vi "Remove Custom Device.vi"(8 "error in":errorcluster, 11 "Ballard ARINC 429 custom device":u64 format="%.0x") -> (0 "error out":errorcluster)   [LabVIEW 2020, in "Ballard ARINC 429 Scripting.lvlib"]
doc: "Removes the specified custom device from the system definition. Once the reference has been removed, it is no longer valid. This VI will return an error if called to remove an invalid reference."
uses:
  Ballard ARINC 429 Scripting.lvlib
  NationalInstruments.VeriStand.SystemDefinitionAPI
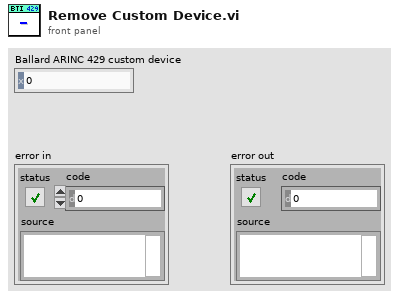
[diagram p1: front panel]
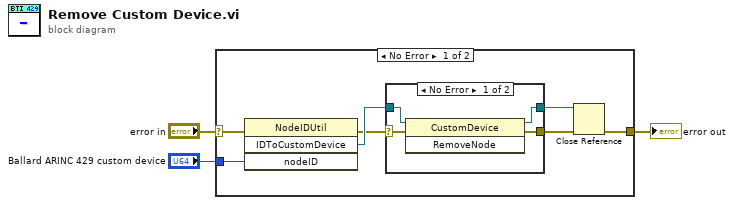
[diagram p0: block diagram]
diagram:
  n1 = case shown="No Error" "error in" {
    selector: "error in" -> [w5 w17]
    tunnel: [w8 w17] -> w2
    tunnel: "Ballard ARINC 429 custom device" -> [w6 _]
    frame No Error {
      n2 = invoke class="NodeIDUtil" method="IDToCustomDevice"(error in=w5, "nodeID"=w6) -> (error out=w4:errorcluster, "IDToCustomDevice"=w7:refnum<k24>)  [unwired: 2 in, 2 out]
      n3 = case shown="No Error" w4 {
        selector: w4 -> [w13 w16]
        tunnel: w7 -> [w14 w15]
        tunnel: [w12 w15] -> w10
        tunnel: [w11 w16] -> w9
        frame No Error {
          n4 = invoke class="CustomDevice" method="RemoveNode"(reference=w14, error in=w13) -> (reference out=w12:refnum<k24>, error out=w11:errorcluster)  [unwired: 1 in, 1 out]
        }
        frame Error {
        }
      }
      n5 = Close Reference(reference=w10, error in (no error)=w9) -> (error out=w8:errorcluster)
    }
    frame Error {
    }
  }
  "error out" <- w2
